vi "Update Property Map Value.vi"(10 "Property data in":T6, 11 "Data Cluster in":T1) -> (3 "Data Cluster out":T1)   [LabVIEW 2020, in "Control Property Tree.lvlib"]
uses:
  Control Property Tree.lvlib
  Module Data--cluster.ctl
  Ctrl Properties Map Data.ctl
  Property array.ctl
  Selected Ctrls - List of Controls.ctl
  Selected Ctrls - List of Properties.ctl
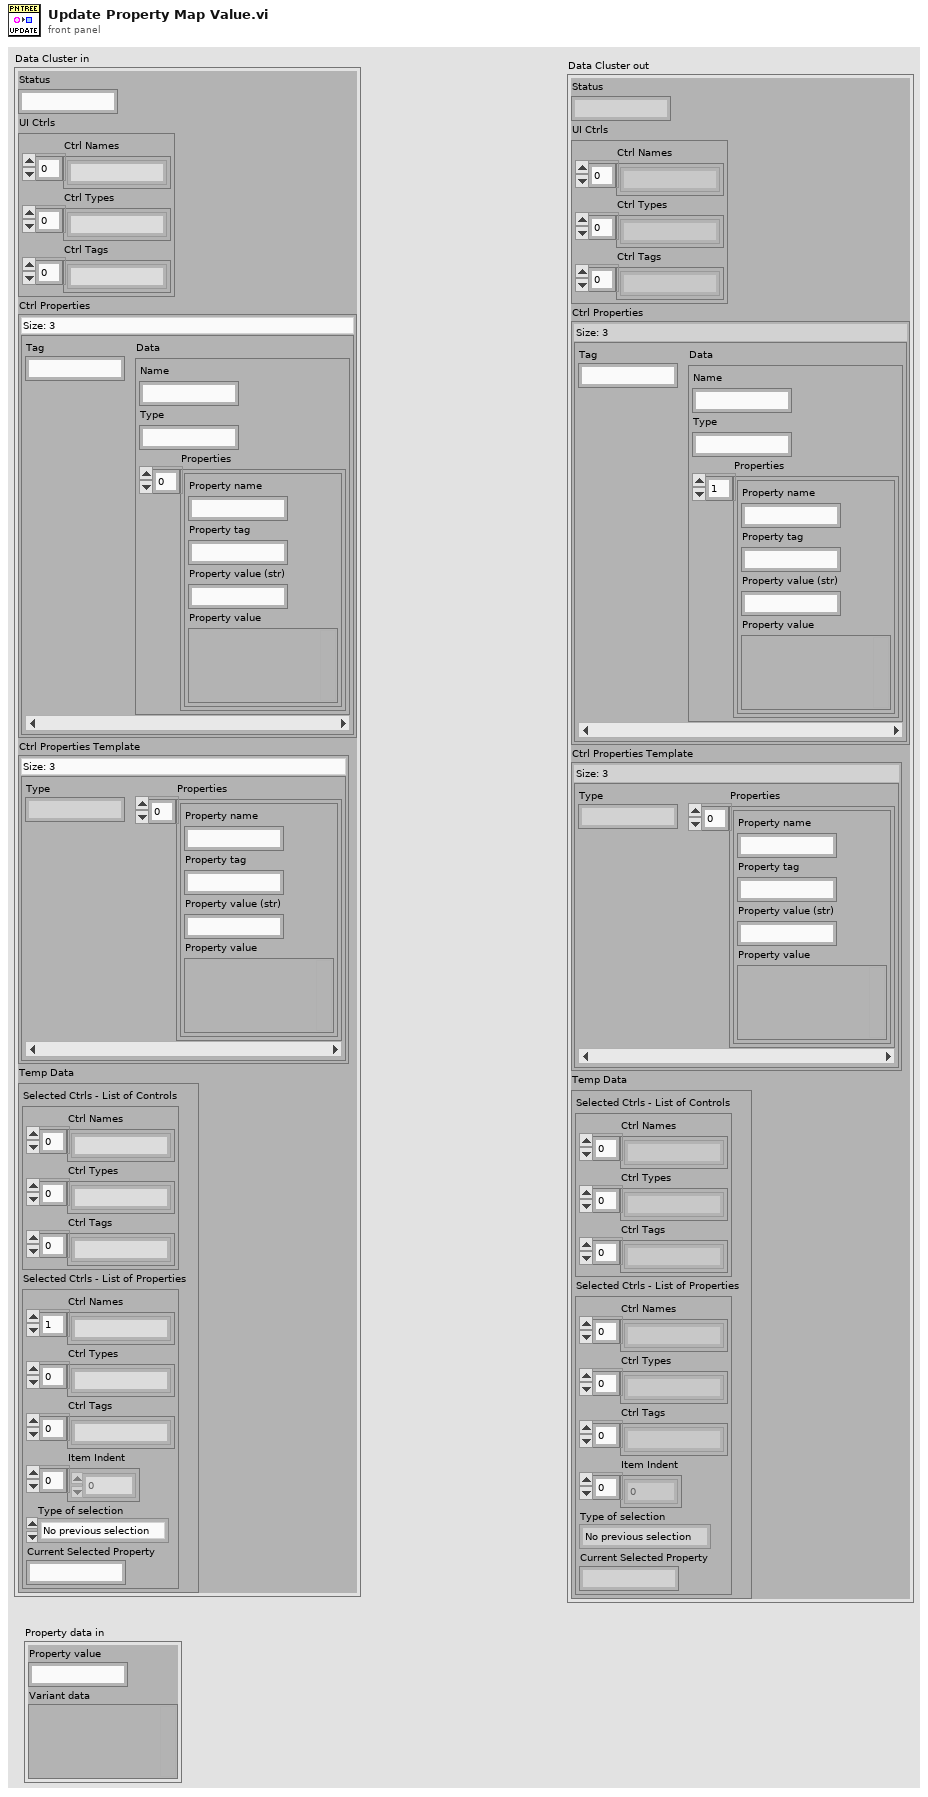
[diagram p1: front panel]
types:
  T1 = typedef "Control Property Tree.lvlib/Module Data--cluster.ctl" = cluster{"Status":string, "UI Ctrls":cluster{"Ctrl Names":string[], "Ctrl Types":string[], "Ctrl Tags":string[]}, "Ctrl Properties":map{string, T2}, "Ctrl Properties Template":map{string, T3}, "Temp Data":cluster{"Selected Ctrls - List of Controls":T4, "Selected Ctrls - List of Properties":T5}}
  T2 = typedef "Control Property Tree.lvlib/Ctrl Properties Map Data.ctl" = cluster{"Name":string, "Type":string, "Properties":T3}
  T3 = typedef "Control Property Tree.lvlib/Property array.ctl" = cluster{"Property name":string, "Property tag":string, "Property value (str)":string, "Property value":variant}[]
  T4 = typedef "Control Property Tree.lvlib/Selected Ctrls - List of Controls.ctl" = cluster{"Ctrl Names":string[], "Ctrl Types":string[], "Ctrl Tags":string[]}
  T5 = typedef "Control Property Tree.lvlib/Selected Ctrls - List of Properties.ctl" = cluster{"Ctrl Names":string[], "Ctrl Types":string[], "Ctrl Tags":string[], "Item Indent":i32[], "Type of selection":enum16{"No previous selection", "Control selected", "Property selected"}, "Current Selected Property":string}
  T6 = cluster{"Property value":string, "Variant data":variant}
  T7 = cluster{"Property name":string, "Property tag":string, "Property value (str)":string, "Property value":variant}
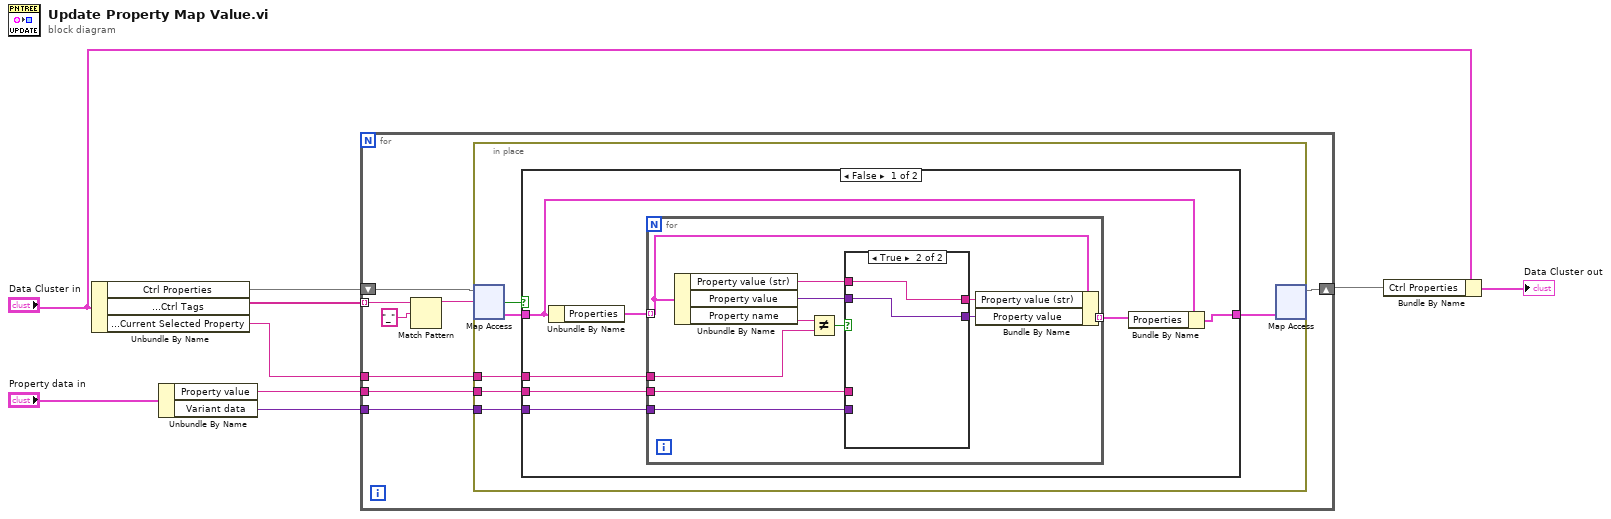
[diagram p0: block diagram]
diagram:
  n1 = Unbundle By Name("Data Cluster in") -> ("Ctrl Properties"=w9:map{string, T2}, "Temp Data.Selected Ctrls - List of Properties.Ctrl Tags"=w8:string[], "Temp Data.Selected Ctrls - List of Properties.Current Selected Property"=w7:string)
  n2 = Unbundle By Name("Property data in") -> ("Property value"=w4:string, "Variant data"=w5:variant)
  n3 = for {
    tunnel: w8 -> [w11] mode=indexing
    tunnel: w7 -> [w16]
    tunnel: w5 -> [w15]
    tunnel: w4 -> [w14]
    shift-right: [w13] -> w2
    shift-left: w9 -> [w17]
    n4 = Match Pattern(string=w11, regular expression="_") -> (before substring=w10:string)  [unwired: 1 in, 3 out]
    n5 = in-place {
      in-place-border: w16 -> [w22]
      in-place-border: w15 -> [w21]
      in-place-border: w14 -> [w18]
      n6 = in-place-map #1(w17, w10) -> (w20:T2, w23:bool)  [unwired: 1 in]
      n7 = case shown="False" w23 {
        tunnel: w20 -> [w26 w46]
        tunnel: w22 -> [w29 _]
        tunnel: w21 -> [w28 _]
        tunnel: [w25 w46] -> w19
        tunnel: w18 -> [w24 _]
        frame False {
          n8 = Unbundle By Name(w26) -> ("Properties"=w30:T3)
          n9 = for {
            tunnel: w30 -> [w39] mode=indexing
            tunnel: w29 -> [w40]
            tunnel: w28 -> [w31]
            tunnel: [w38] -> w27 mode=indexing
            tunnel: w24 -> [w32]
            n10 = Unbundle By Name(w39) -> ("Property value (str)"=w35:string, "Property value"=w33:variant, "Property name"=w41:string)
            n11 = Not Equal?(x=w41, y=w40) -> (x != y?=w37:bool)
            n12 = case shown="True" w37 {
              tunnel: [w43 w45] -> w36
              tunnel: w35 -> [_ w45]
              tunnel: [w42 w44] -> w34
              tunnel: w33 -> [_ w44]
              tunnel: w32 -> [w43 _]
              tunnel: w31 -> [w42 _]
              frame False {
              }
              frame True {
              }
            }
            n13 = Bundle By Name(cluster=w39, "Property value (str)"=w36, "Property value"=w34) -> (w38:T7)
          }
          n14 = Bundle By Name(cluster=w26, "Properties"=w27) -> (w25:T2)
        }
        frame True {
        }
      }
      n15 = in-place-map #1(w19) -> (w13:map{string, T2})  [unwired: 1 in, 2 out]
    }
  }
  n16 = Bundle By Name(cluster="Data Cluster in", "Ctrl Properties"=w2) -> (→"Data Cluster out":T1)
